vi "SV TDMS Read XY (1 Ch).vi"(0 "tdms file":refnum<k34>, 5 "group name in":string="XY", 7 "channel name in":string="Channel0", 11 "error in":errorcluster) -> (3 "scale labels":T2, 4 "tdms file out":refnum<k34>, 6 "group name out":string, 8 "channel name out":string, 10 "XY":cluster{"X":dbl[], "Y":dbl[]}, 13 "unit info":T1, 15 "error out":errorcluster)   [LabVIEW 2017]
uses:
  <vilib>/addons/_NISVFA/_Shared subVIs/Controls/NI Channel Properties.ctl
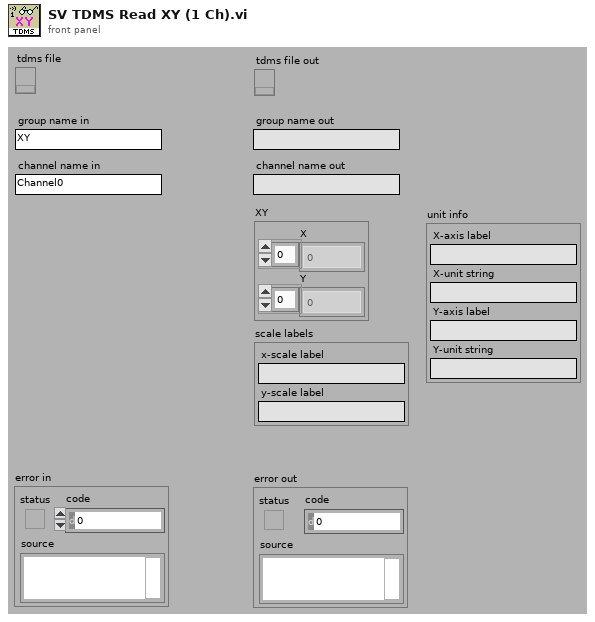
[diagram p1: front panel]
types:
  T1 = cluster{"X-axis label":string, "X-unit string":string, "Y-axis label":string, "Y-unit string":string}
  T2 = cluster{"x-scale label":string, "y-scale label":string}
  T3 = typedef "NI Channel Properties.ctl" = u16
  T4 = cluster{"scale label with units":string, "scale label with units":string}
  T5 = cluster{"X-axis label":string, "X-axis label":string, "X-axis label":string, "X-axis label":string}
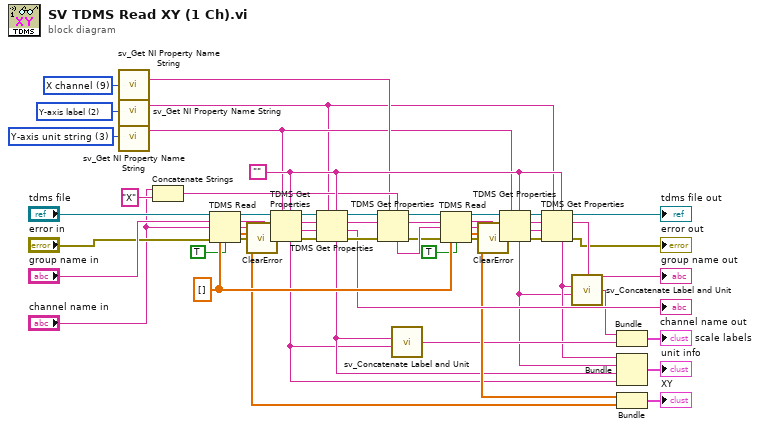
[diagram p0: block diagram]
diagram:
  w36 = T3 3 items=["Channel name", "Channel description", "Y-axis label", "Y-axis unit string", "X-axis label", "X-axis unit string", "x0", "dx", "Number of samples", "X channel", "Filter settled", "dB reference", "Window", "Window parameter", "Window size", "FFT size", "Peak units", "Spectrum type", "Magnitude scale", "Spectral density", "Sensor sensitivity (mV/EU)", "X-axis domain", "LabVIEW datatype"] ("property")
  w37 = T3 2 items=["Channel name", "Channel description", "Y-axis label", "Y-axis unit string", "X-axis label", "X-axis unit string", "x0", "dx", "Number of samples", "X channel", "Filter settled", "dB reference", "Window", "Window parameter", "Window size", "FFT size", "Peak units", "Spectrum type", "Magnitude scale", "Spectral density", "Sensor sensitivity (mV/EU)", "X-axis domain", "LabVIEW datatype"] ("property")
  w39 = T3 9 items=["Channel name", "Channel description", "Y-axis label", "Y-axis unit string", "X-axis label", "X-axis unit string", "x0", "dx", "Number of samples", "X channel", "Filter settled", "dB reference", "Window", "Window parameter", "Window size", "FFT size", "Peak units", "Spectrum type", "Magnitude scale", "Spectral density", "Sensor sensitivity (mV/EU)", "X-axis domain", "LabVIEW datatype"] ("property")
  w44 = "" ("X-axis label")
  w30 = dbl[] [] ("X")
  n1 = call <vilib>:"sv_Get NI Property Name String.vi"("property"=w39) -> ("TDMS property name"=w38:string)  [unwired: 13 in, 1 out]
  n2 = call <vilib>:"sv_Get NI Property Name String.vi"("property"=w37) -> ("TDMS property name"=w34:string)  [unwired: 13 in, 1 out]
  n3 = call <vilib>:"sv_Get NI Property Name String.vi"("property"=w36) -> ("TDMS property name"=w35:string)  [unwired: 13 in, 1 out]
  n4 = Concatenate Strings("channel name in", "X" ("string")) -> (w40:string)
  n5 = TDMS Read(0:"tdms file", 5:"group name in", 7:"channel name in", 11:"error in", 12:w30, 13:TRUE ("return channels in file order? (F)")) -> (4:w51:refnum<k34>, 6:w16:string, 8:w19:string, 10:w20:dbl[], 15:w3:errorcluster)  [unwired: 2 in, 1 out]
  n6 = call <vilib>:"ClearError.vi"("error in (no error)"=w3) -> ("error out"=w47:errorcluster)
  n7 = TDMS Get Properties(5:w44, 7:w35, 8:w47, 9:w19, 10:w16, 11:w51) -> (0:w46:errorcluster, 1:w50:string, 2:w49:string, 3:w45:refnum<k34>, 4:w7:string)  [unwired: 1 out]
  n8 = TDMS Get Properties(5:w44, 7:w34, 8:w46, 9:w50, 10:w49, 11:w45) -> (0:w43:errorcluster, 1:→"channel name out":string, 2:w42:string, 3:w41:refnum<k34>, 4:w8:string)  [unwired: 1 out]
  n9 = TDMS Get Properties(5:w40, 7:w38, 8:w43, 10:w42, 11:w41) -> (0:w26:errorcluster, 2:w28:string, 3:w29:refnum<k34>, 4:w27:string)  [unwired: 1 in, 2 out]
  n10 = call <vilib>:"sv_Concatenate Label and Unit.vi"("unit string"=w7, "label"=w8) -> ("scale label with units"=w13:string)  [unwired: 4 in]
  n11 = TDMS Read(0:w29, 5:w28, 7:w27, 11:w26, 12:w30, 13:TRUE ("return channels in file order? (F)")) -> (4:w54:refnum<k34>, 6:w17:string, 8:w18:string, 10:w21:dbl[], 15:w4:errorcluster)  [unwired: 2 in, 1 out]
  n12 = call <vilib>:"ClearError.vi"("error in (no error)"=w4) -> ("error out"=w55:errorcluster)
  n13 = TDMS Get Properties(5:w44, 7:w35, 8:w55, 9:w18, 10:w17, 11:w54) -> (0:w5:errorcluster, 1:w52:string, 2:w53:string, 4:w9:string)  [unwired: 2 out]
  n14 = TDMS Get Properties(5:w44, 7:w34, 8:w5, 9:w52, 10:w53, 11:w54) -> (0:→"error out":errorcluster, 2:→"group name out":string, 3:→"tdms file out":refnum<k34>, 4:w10:string)  [unwired: 2 out]
  n15 = call <vilib>:"sv_Concatenate Label and Unit.vi"("unit string"=w9, "label"=w10) -> ("scale label with units"=w14:string)  [unwired: 4 in]
  n16 = Bundle("scale label with units"=w14, "scale label with units"=w13) -> (→"scale labels":T4)  [unwired: 1 in]
  n17 = Bundle("X-axis label"=w10, "X-axis label"=w9, "X-axis label"=w8, "X-axis label"=w7) -> (→"unit info":T5)  [unwired: 1 in]
  n18 = Bundle("X"=w21, "X"=w20) -> (→"XY":cluster{"X":dbl[], "X":dbl[]})  [unwired: 1 in]
